vi "Read LUT.vi"(8 "error in (no error)":errorcluster, 11 "ObjectLUT in":refnum<class "ObjectLUT.lvclass">) -> (0 "error out":errorcluster, 2 "LUT":variant, 3 "ObjectLUT out":refnum<class "ObjectLUT.lvclass">)   [LabVIEW 2020, in "ORM_lib.lvlib" / "ObjectLUT.lvclass"]
uses:
  ObjectLUT.lvclass
  ObjectLUT.lvclass/ObjectLUT.ctl
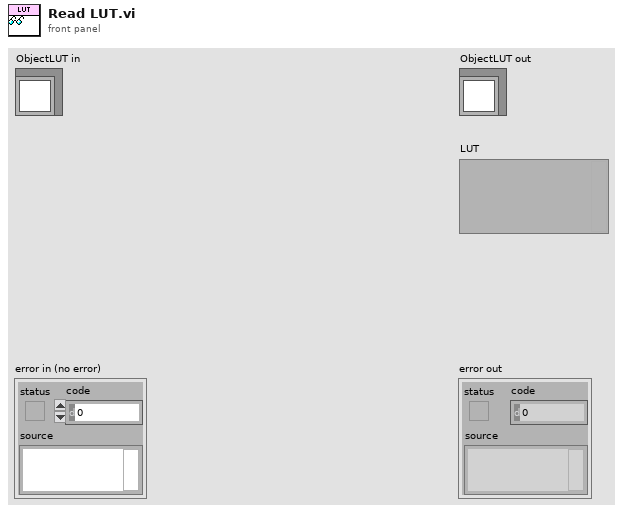
[diagram p1: front panel]
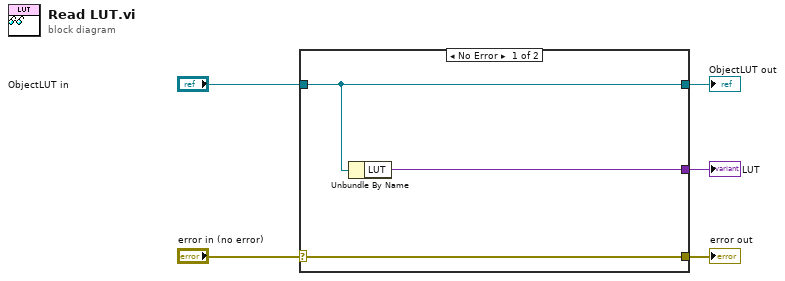
[diagram p0: block diagram]
diagram:
  n1 = case shown="No Error" "error in (no error)" {
    selector: "error in (no error)" -> [w8 w9]
    tunnel: [w8 w9] -> w4
    tunnel: [w7 w10] -> w2
    tunnel: "ObjectLUT in" -> [w7 w10]
    tunnel: [w6 _] -> w1
    frame No Error {
      n2 = Unbundle By Name(w7) -> ("LUT"=w6:variant)
    }
    frame Error {
    }
  }
  "error out" <- w4
  "ObjectLUT out" <- w2
  "LUT" <- w1
